vi "사인파형(SubVI).vi"() -> (0 "경로":path, 1 "웨이브폼 그래프":dbl[](graph))   [LabVIEW 2014]
uses:
  <vilib>/Utility/file.llb/Write To Spreadsheet File (DBL).vi
  <vilib>/Analysis/NI_AALBase.lvlib
panel:
  in  "Cancel":bool
  in  "OK":bool
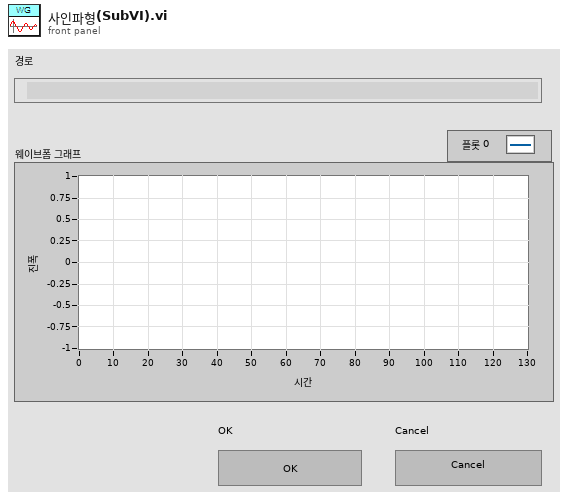
[diagram p1: front panel]
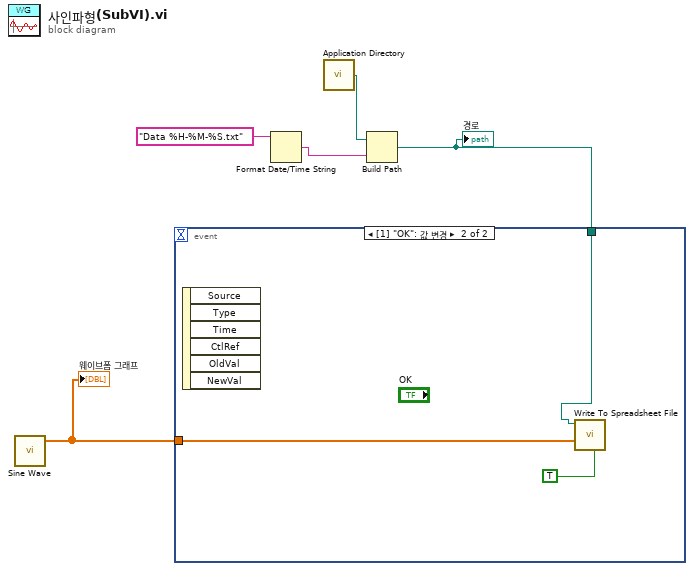
[diagram p0: block diagram]
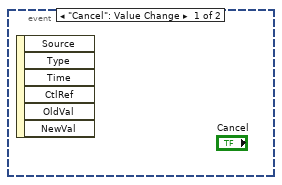
[diagram p2: hidden frame]
diagram:
  n1 = call <vilib>:"Sine Wave.vi"() -> ("sine wave"=w5:dbl[])  [unwired: 5 in, 2 out]
  "웨이브폼 그래프" <- w5
  n2 = Format Date/Time String(time format string (%c)="Data %H-%M-%S.txt" ("시간 포맷 문자열 (%c)")) -> (date/time string=w4:string)  [unwired: 2 in]
  n3 = call <vilib>:"Application Directory.vi"() -> ("Application Directory"=w3:path)
  n4 = Build Path(base path=w3, name or relative path=w4) -> (appended path=w1:path)
  "경로" <- w1
  n5 = event shown="[1] \"OK\": 값 변경" {
    selector: _ -> [_ _]
    dyn-events: _ -> [_ _]
    timeout: _ -> [_ _]
    tunnel: w5 -> [_ w7]
    tunnel: w1 -> [_ w6]
    event "Cancel": Value Change {
      n6 = event-data() -> ()  [unwired: 1 in, 6 out]
    }
    event "OK": Value Change {
      n7 = event-data() -> ()  [unwired: 1 in, 6 out]
      n8 = call-poly <vilib>:"Write To Spreadsheet File.vi"("transpose? (no:F)"=TRUE, "1D data"=w7, "file path (dialog if empty)"=w6) -> ()  [unwired: 5 in, 1 out]
    }
  }
